vi "ultrasonic sensor test.vi"   [LabVIEW 2010, in "Test1.lvrbt"]
uses:
  Test1.lvrbt
  <vilib>/NXT/Subs/MotorOutput.ctl
  <vilib>/NXT/Block Support/NXT_InputPort.ctl
  <vilib>/NXT/Dual Mode Library/Motors/MotorReverse.vi
  <vilib>/NXT/Dual Mode Library/Waits/Wait_Further.vi
  <vilib>/NXT/Dual Mode Library/Motors/MotorCoast.vi
types:
  T1 = typedef "NXT_InputPort.ctl" = u8
  T2 = typedef "MotorOutput.ctl" = u8
  T3 = typedef "LVHSConnector.ctl" = cluster{"Hardware":string, "Flattened String":string}
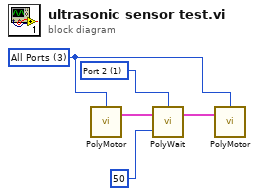
[diagram p0: block diagram]
diagram:
  w3 = T1 1 items=["Port 1", "Port 2", "Port 3", "Port 4"] ("Port (Port 1)")
  w2 = T2 3 items=["Port A", "Port B", "Port C", "All Ports"] ("Output Port (All Ports)")
  n1 = call-poly <vilib>:"PolyMotor.vi"("Output Port (All Ports)"=w2) -> ("NXT"=w5:T3)  [unwired: 3 in]
  n2 = call-poly <vilib>:"PolyWait.vi"("Distance (40)"=i16 50, "NXT"=w5, "Port (Port 4)"=w3) -> ("NXT"=w4:T3)  [unwired: 1 in]
  n3 = call-poly <vilib>:"PolyMotor.vi"("NXT"=w4, "Port (All Ports)"=w2) -> ()  [unwired: 2 in, 1 out]
